vi "AeroFlowSanitise.vi"(6 "ReductionCode":i32[](array[numeric]), 11 "Raw\n   Vmag         U             V             W          Cone":dbl[][](array[numeric]) caption="RawReducedData") -> (0 "nGoodAF":i16, 2 "CleanOutput":T1)   [LabVIEW 2016]
doc: "Removes points where any component is NaN or there was a reduction error. Includes an ouput array of Xvals, to allow plotting to a common X-axis with pressures."
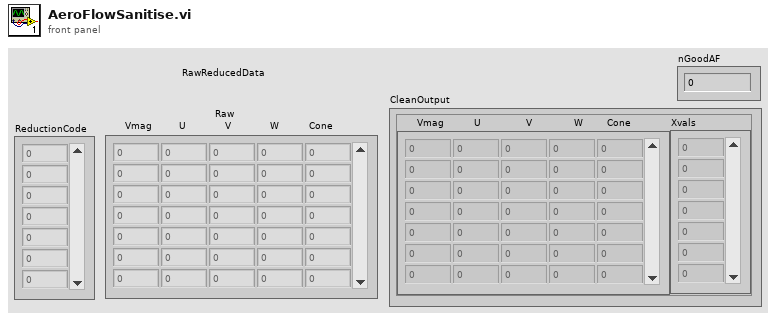
[diagram p1: front panel]
types:
  T1 = cluster{"   Vmag          U               V              W        Cone":dbl[][], "Xvals":i32[]}
  T2 = cluster{"Raw\n   Vmag         U             V             W          Cone":dbl[][], i32[]}
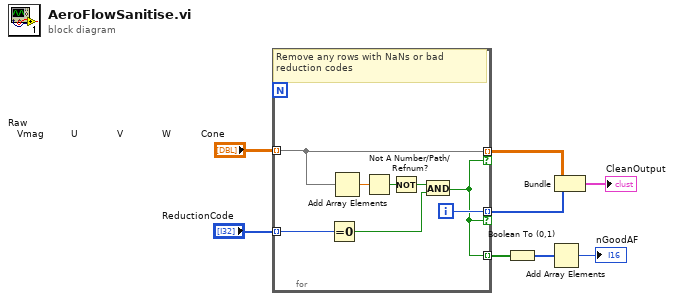
[diagram p0: block diagram]
diagram:
  n1 = for {
    tunnel: "Raw\n   Vmag         U             V             W          Cone" -> [w15] mode=indexing
    tunnel: [w15] -> w3 mode=indexing if=w9
    tunnel: [w13] -> w2 mode=indexing if=w9
    tunnel: "ReductionCode" -> [w11] mode=indexing
    tunnel: [w9] -> w6 mode=indexing
    i -> [w13]
    # "Remove any rows with NaNs or bad reduction codes"
    n2 = Equal To 0?(x=w11) -> (x = 0?=w10:bool)
    n3 = Add Array Elements(numeric array=w15) -> (sum=w16:dbl)
    n4 = Not A Number/Path/Refnum?(number/path/refnum=w16) -> (NaN/Path/Refnum?=w14:bool)
    n5 = Not(x=w14) -> (.not. x?=w12:bool)
    n6 = And(x=w12, y=w10) -> (x .and. y?=w9:bool)
  }
  n7 = Boolean To (0,1)(Boolean=w6) -> (0, 1=w5:i16[])
  n8 = Add Array Elements(numeric array=w5) -> (sum=→"nGoodAF":i16)
  n9 = Bundle("Raw\n   Vmag         U             V             W          Cone"=w3, w2) -> (→"CleanOutput":T2)  [unwired: 1 in]
